vi "Find All Partial With Levelss.vi"(9 "Level":i32, 10 "Name":string, 11 "Tree":variant) -> (0 "Found?":bool, 1 "Levels":i32[](array[numeric]), 2 "Match":variant[](array[variant]), 3 "Node Name":string[](array[string]))   [LabVIEW 2019, in "Tree.lvclass"]
uses:
  Tree.lvclass
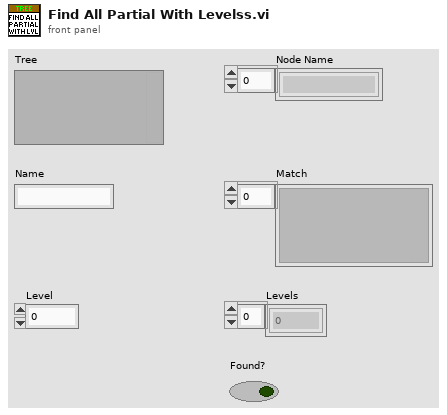
[diagram p1: front panel]
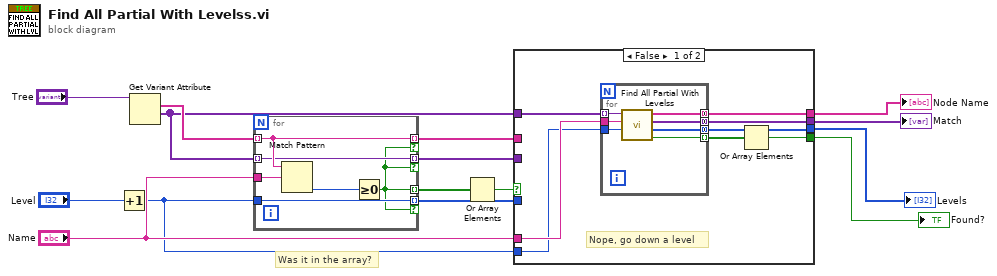
[diagram p0: block diagram]
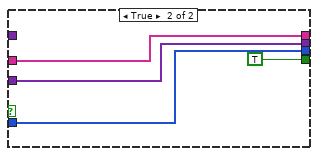
[diagram p2: hidden frame]
diagram:
  # "Was it in the array?"
  n1 = Increment(x="Level") -> (x+1=w1:i32)
  n2 = Get Variant Attribute(Variant="Tree") -> (names=w12:string[], values=w11:variant[])  [unwired: 3 in, 2 out]
  n3 = for {
    tunnel: w12 -> [w19] mode=indexing
    tunnel: "Name" -> [w21]
    tunnel: [w19] -> w9 mode=indexing if=w16
    tunnel: [w16] -> w6 mode=indexing
    tunnel: w11 -> [w18] mode=indexing
    tunnel: [w18] -> w8 mode=indexing if=w16
    tunnel: w1 -> [w17]
    tunnel: [w17] -> w3 mode=indexing if=w16
    n4 = Match Pattern(string=w19, regular expression=w21) -> (offset past match=w20:i32)  [unwired: 1 in, 3 out]
    n5 = Greater Or Equal To 0?(x=w20) -> (x >= 0?=w16:bool)
  }
  n6 = Or Array Elements(Boolean array=w6) -> (logical OR=w5:bool)
  n7 = case shown="False" w5 {
    tunnel: "Name" -> [w29 _]
    tunnel: w11 -> [w27 _]
    tunnel: [w28 w39] -> w14
    tunnel: [w22 TRUE ("Found?")] -> w13
    tunnel: w9 -> [_ w38]
    tunnel: w8 -> [_ w39]
    tunnel: [w26 w38] -> w7
    tunnel: w3 -> [_ w37]
    tunnel: [w24 w37] -> w2
    tunnel: w1 -> [w25 _]
    frame False {
      # "Nope, go down a level"
      n8 = for {
        tunnel: w27 -> [w36] mode=indexing
        tunnel: w29 -> [w33]
        tunnel: [w34] -> w28 mode=concatenating
        tunnel: [w30] -> w23 mode=indexing
        tunnel: [w35] -> w26 mode=concatenating
        tunnel: w25 -> [w32]
        tunnel: [w31] -> w24 mode=concatenating
        n9 = call "Find All Partial With Levelss.vi"("Level"=w32, "Name"=w33, "Tree"=w36) -> ("Found?"=w30:bool, "Levels"=w31:i32[], "Match"=w34:variant[], "Node Name"=w35:string[])  [unwired: 5 in]
      }
      n10 = Or Array Elements(Boolean array=w23) -> (logical OR=w22:bool)
    }
    frame True {
    }
  }
  "Found?" <- w13
  "Match" <- w14
  "Node Name" <- w7
  "Levels" <- w2
